vi "commutation.vi"(9 "Hall C":bool, 10 "Hall B":bool, 11 "Hall A":bool) -> (3 "Commutation":i32)   [LabVIEW 2020]
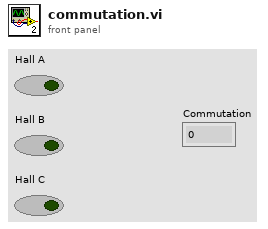
[diagram p1: front panel]
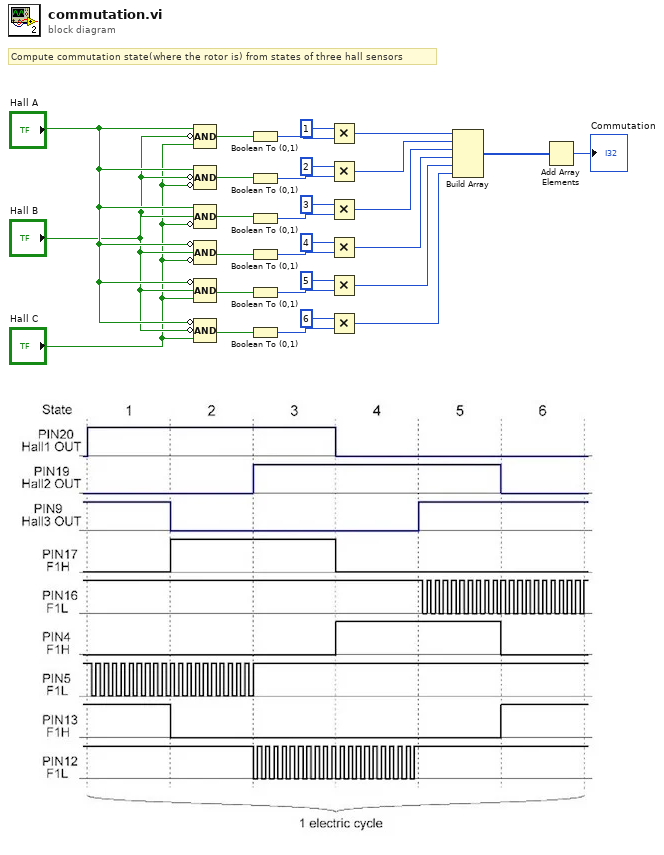
[diagram p0: block diagram]
diagram:
  # "Compute commutation state(where the rotor is) from states of three hall sensors"
  n1 = Compound Arithmetic op=AND("Hall A", invert "Hall B", "Hall C") -> (w29:bool)
  n2 = Compound Arithmetic op=AND("Hall A", invert "Hall B", invert "Hall C") -> (w21:bool)
  n3 = Compound Arithmetic op=AND("Hall A", "Hall B", invert "Hall C") -> (w22:bool)
  n4 = Compound Arithmetic op=AND(invert "Hall A", "Hall B", invert "Hall C") -> (w18:bool)
  n5 = Compound Arithmetic op=AND(invert "Hall A", "Hall B", "Hall C") -> (w15:bool)
  n6 = Compound Arithmetic op=AND(invert "Hall A", invert "Hall B", "Hall C") -> (w12:bool)
  n7 = Boolean To (0,1)(Boolean=w29) -> (0, 1=w27:i16)
  n8 = Boolean To (0,1)(Boolean=w21) -> (0, 1=w25:i16)
  n9 = Boolean To (0,1)(Boolean=w22) -> (0, 1=w23:i16)
  n10 = Boolean To (0,1)(Boolean=w18) -> (0, 1=w19:i16)
  n11 = Boolean To (0,1)(Boolean=w15) -> (0, 1=w16:i16)
  n12 = Boolean To (0,1)(Boolean=w12) -> (0, 1=w13:i16)
  n13 = Multiply(x=1, y=w27) -> (x*y=w8:i32)
  n14 = Multiply(x=2, y=w25) -> (x*y=w7:i32)
  n15 = Multiply(x=3, y=w23) -> (x*y=w6:i32)
  n16 = Multiply(x=4, y=w19) -> (x*y=w5:i32)
  n17 = Multiply(x=5, y=w16) -> (x*y=w1:i32)
  n18 = Multiply(x=6, y=w13) -> (x*y=w4:i32)
  n19 = Build Array(w8, w7, w6, w5, w1, w4) -> (w3:i32[])
  n20 = Add Array Elements(numeric array=w3) -> (sum=→"Commutation":i32)
